vi "Remote-Read_Api.vi"() -> ()   [LabVIEW 2019]
uses:
  Controller/F710PackedLibrary.lvlibp/stick.ctl
  Controller/F710PackedLibrary.lvlibp
panel:
  out "S-BUS Controller":T2 {"CH16" scale=-1024.0..1024.0; "CH15" scale=-1024.0..1024.0; "CH14" scale=-1024.0..1024.0; "CH13" scale=-1024.0..1024.0; "CH12" scale=-1024.0..1024.0; "CH11" scale=-1024.0..1024.0; "CH10" scale=-1024.0..1024.0; "CH9" scale=-1024.0..1024.0; "CH8" scale=-1024.0..1024.0; "CH7" scale=-1024.0..1024.0; "CH6" scale=-1024.0..1024.0; "CH5" scale=-1024.0..1024.0}
  out "error out":errorcluster
  in  "error in (no error)":errorcluster
  in  "停止讀值":bool
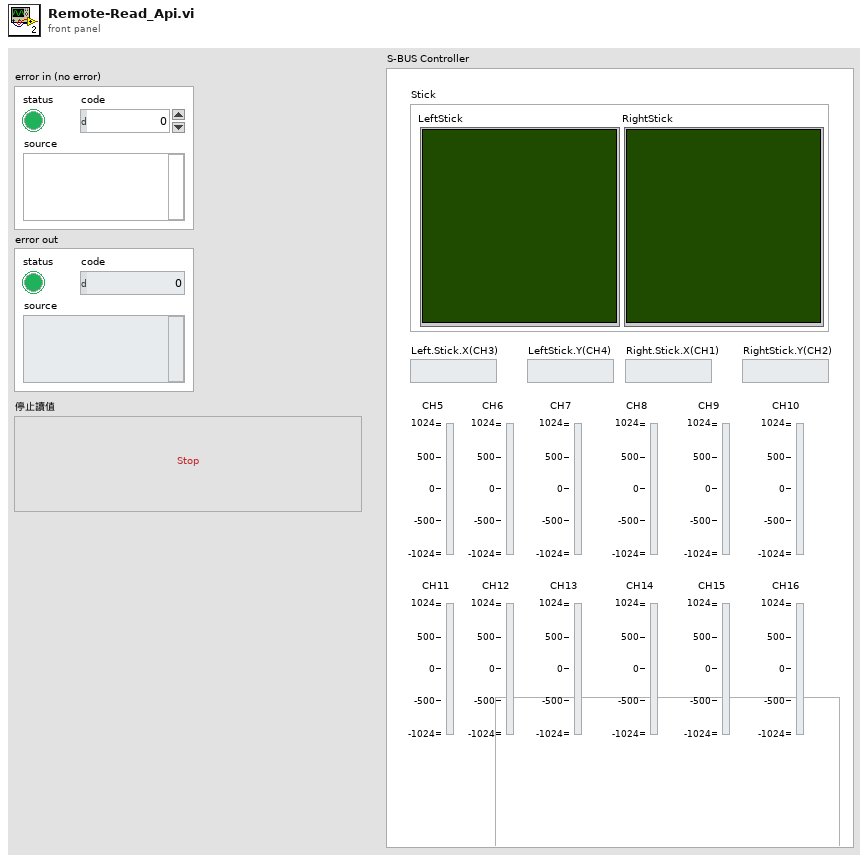
[diagram p1: front panel]
types:
  T1 = typedef "F710PackedLibrary.lvlibp/stick.ctl" = cluster{"X":dbl, "Y":dbl}[]
  T2 = cluster{"Stick":cluster{"LeftStick":T1, "RightStick":T1}, "Left.Stick.X(CH3)":dbl, "LeftStick.Y(CH4)":dbl, "Right.Stick.X(CH1)":dbl, "RightStick.Y(CH2)":dbl, "CH5":dbl, "CH6":dbl, "CH7":dbl, "CH8":dbl, "CH9":dbl, "CH10":dbl, "CH11":dbl, "CH12":dbl, "CH13":dbl, "CH14":dbl, "CH15":dbl, "CH16":dbl}
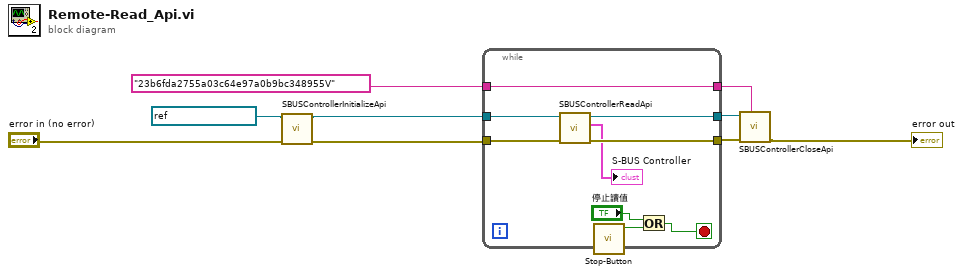
[diagram p0: block diagram]
diagram:
  n1 = call "SBUSControllerInitializeApi.vi"("error in (no error)"="error in (no error)", "VISA Refnum in"=refnum<visa-resource-name> "ASRL2::INSTR") -> ("error out"=w2:errorcluster, "VISA Refnum out"=w8:refnum<visa-resource-name>)  [unwired: 8 in]
  n2 = while {
    tunnel: "23b6fda2755a03c64e97a0b9bc348955V" ("設備授權碼") -> [w15]
    tunnel: [w15] -> w7
    tunnel: w8 -> [w12]
    tunnel: [w11] -> w4
    tunnel: w2 -> [w13]
    tunnel: [w14] -> w5
    stop <- w16 stop-if-true
    n3 = call "SBUSControllerReadApi.vi"("error in (no error)"=w13, "VISA Refnum in"=w12) -> ("error out"=w14:errorcluster, "S-BUS Controller"=→"S-BUS Controller":T2, "VISA Refnum out"=w11:refnum<visa-resource-name>)  [unwired: 7 in]
    n4 = call "Stop-Button.vi"() -> ("顯示按下?"=w18:bool)  [unwired: 10 in, 1 out]
    n5 = Or(x="停止讀值", y=w18) -> (x .or. y?=w16:bool)
  }
  n6 = call "SBUSControllerCloseApi.vi"("設備授權碼"=w7, "error in (no error)"=w5, "VISA Refnum in"=w4) -> ("error out"=→"error out":errorcluster)  [unwired: 8 in]
